vi "calculator.vi"() -> ()   [LabVIEW 2019]
panel:
  out "Boolean 2":bool
  out "Boolean":bool
  in  "Slide 2":dbl(slide) scale=0.0..100.0
  in  "Slide":dbl(slide) scale=0.0..100.0
  out "Numeric 3":dbl
  out "Numeric 2":dbl
  out "Numeric":dbl
  out "Tank":dbl(slide) scale=0.0..300.0
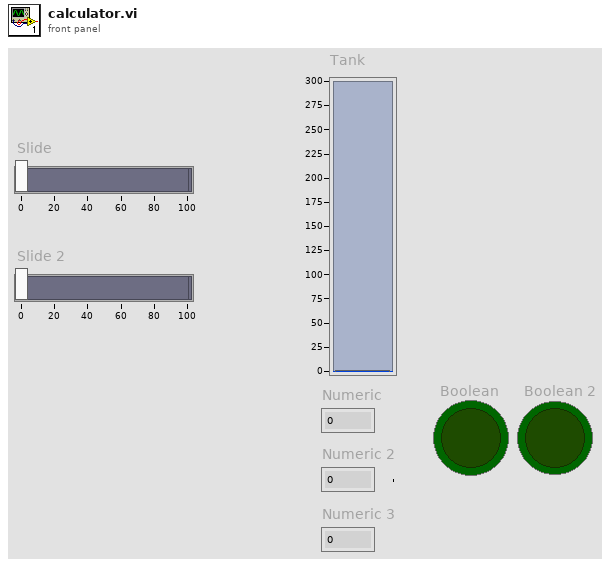
[diagram p1: front panel]
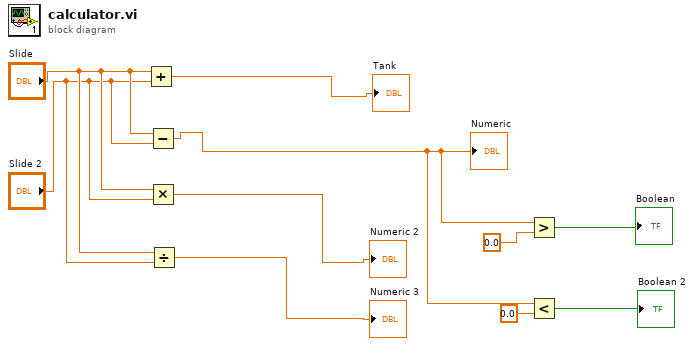
[diagram p0: block diagram]
diagram:
  n1 = Add(x="Slide", y="Slide 2") -> (x+y=→"Tank":dbl)
  n2 = Subtract(x="Slide", y="Slide 2") -> (x-y=w3:dbl)
  "Numeric" <- w3
  n3 = Multiply(x="Slide", y="Slide 2") -> (x*y=→"Numeric 2":dbl)
  n4 = Divide(x="Slide", y="Slide 2") -> (x/y=→"Numeric 3":dbl)
  n5 = Greater?(x=w3, y=0.0) -> (0:→"Boolean":bool)
  n6 = Less?(x=w3, y=0.0) -> (x < y?=→"Boolean 2":bool)
